vi "Reduction_stop.vi"() -> ()   [LabVIEW 2021]
panel:
  out "Reduction_stop":bool
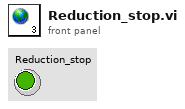
[diagram p1: front panel]
diagram:
